vi "wrap_string (SubVI).vi"(11 "in":string) -> (3 "String":string)   [LabVIEW 2014]
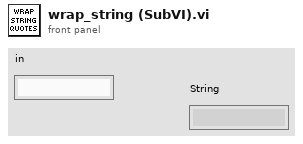
[diagram p1: front panel]
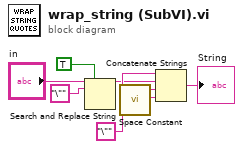
[diagram p0: block diagram]
diagram:
  w5 = "\"" ("string")
  n1 = Search and Replace String(replace all?=TRUE ("replace all? (F)"), input string="in", search string="\"") -> (result string=w3:string)  [unwired: 5 in, 3 out]
  n2 = call <vilib>:"Space Constant.vi"() -> ("String"=w7:string)
  n3 = Concatenate Strings(w5, w3, w5, w7) -> (→"String":string)
